vi "27-type_type.vi"(3 "this":i32, 4 "count in":i32, 5 "button":i32, 6 "Cluster":T1={"Auto1"=TRUE, "Auto2"=TRUE, "Rel1"=FALSE, "Rel2"=FALSE, "Filt1"=FALSE, "Filt2"=FALSE, "Rate"=enum."Slow", "Range1"=enum."10mV", "Range2"=enum."100mV", "Filt3"=FALSE, "Filt4"=FALSE, "Rel temp 1"=FALSE, "Analog1"=FALSE, "Analog2"=FALSE, "Analog temp 1"=FALSE, "Digital1"=FALSE, "Digital2"=FALSE, "Digital temp 1 "=FALSE, "Window1"=enum."None", "Window2"=enum."None", "Window temp 1"=enum."None", "RDGS1"="010", "RDGS2"="010", "RDGS temp 1"="010", "Type_type1"=TRUE, "Type_type2"=TRUE, "Type_type temp 1"=TRUE, "LSync"=FALSE, "Unit"=enum."C", "Sens"=TRUE, "Type tcoupl"=enum."J", "Junc"=TRUE, "prevState"=0, "Rel temp 2"=FALSE, "Analog temp 2"=FALSE, "Digital temp 2"=FALSE, "Type_type temp 2"=TRUE, "RDGS temp 2"="010", "Window temp 2"=enum."None", "address"="0"}) -> (0 "next state":i32, 1 "count out":i32, 2 "Cluster 2":T1)   [LabVIEW 2017]
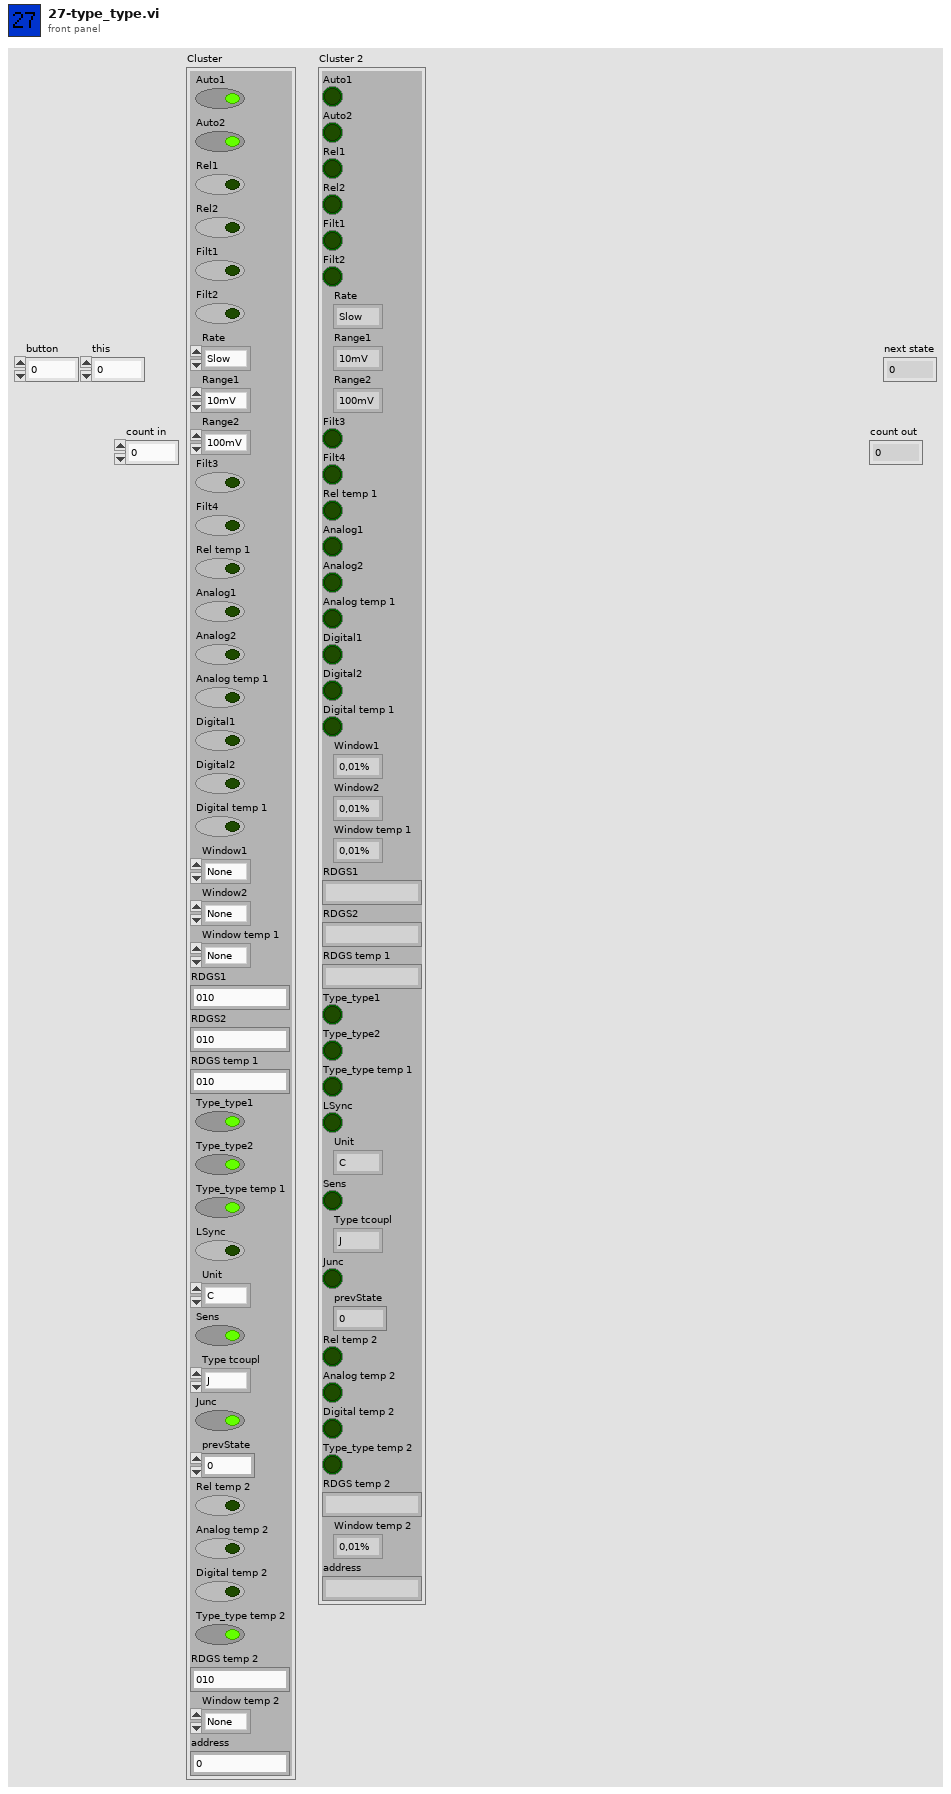
[diagram p1: front panel]
types:
  T1 = cluster{"Auto1":bool, "Auto2":bool, "Rel1":bool, "Rel2":bool, "Filt1":bool, "Filt2":bool, "Rate":enum16{"Slow", "Fast", "Med"}, "Range1":enum16{"10mV", "100mV", "1V", "10V", "100V"}, "Range2":enum16{"100mV", "1V", "10V"}, "Filt3":bool, "Filt4":bool, "Rel temp 1":bool, "Analog1":bool, "Analog2":bool, "Analog temp 1":bool, "Digital1":bool, "Digital2":bool, "Digital temp 1 ":bool, "Window1":enum16{"0,01%", "0,1%", "1%", "10%", "None"}, "Window2":enum16{"0,01%", "0,1%", "1%", "10%", "None"}, "Window temp 1":enum16{"0,01%", "0,1%", "1%", "10%", "None"}, "RDGS1":string, "RDGS2":string, "RDGS temp 1":string, "Type_type1":bool, "Type_type2":bool, "Type_type temp 1":bool, "LSync":bool, "Unit":enum16{"C", "K", "F"}, "Sens":bool, "Type tcoupl":enum16{"J", "K", "T", "E", "R", "S", "B", "N"}, "Junc":bool, "prevState":i32, "Rel temp 2":bool, "Analog temp 2":bool, "Digital temp 2":bool, "Type_type temp 2":bool, "RDGS temp 2":string, "Window temp 2":enum16{"0,01%", "0,1%", "1%", "10%", "None"}, "address":string}
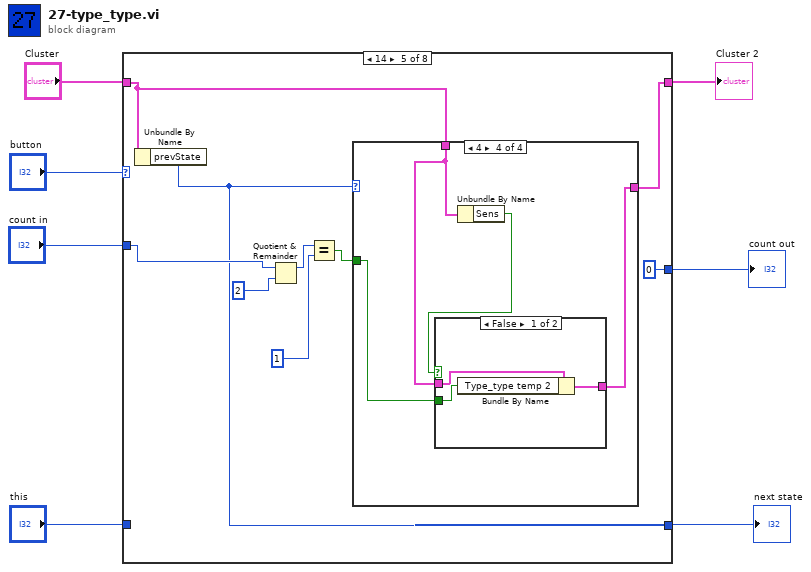
[diagram p0: block diagram]
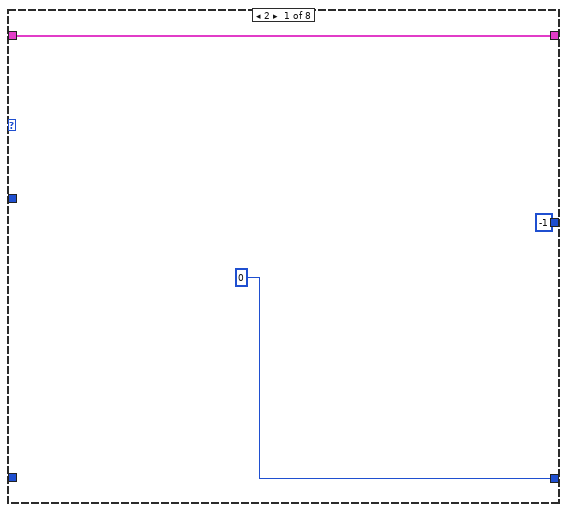
[diagram p2: hidden frame]
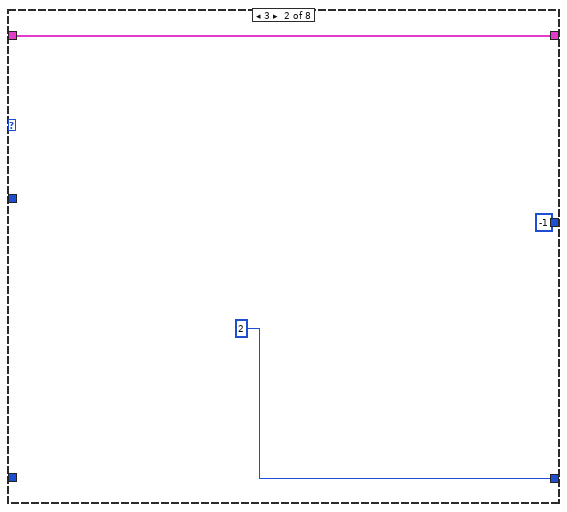
[diagram p3: hidden frame]
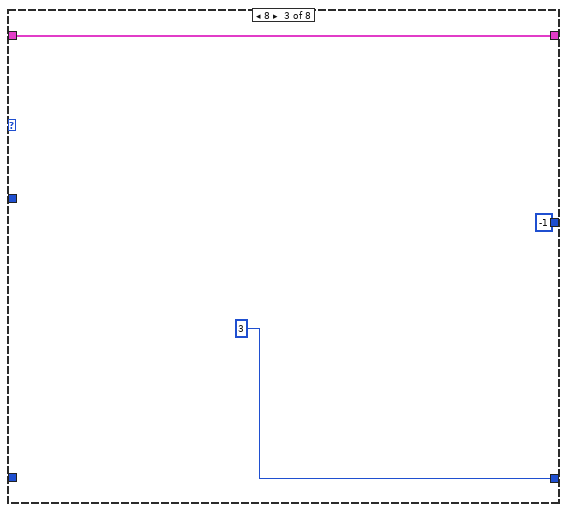
[diagram p4: hidden frame]
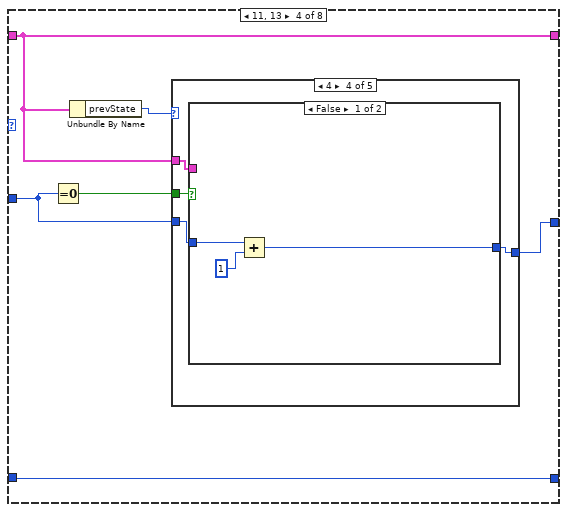
[diagram p5: hidden frame]
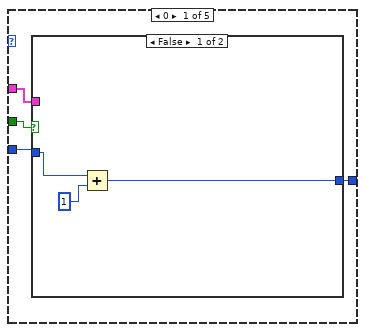
[diagram p6: hidden frame]
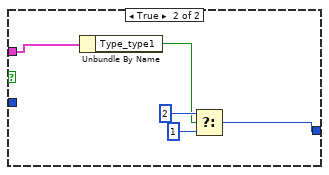
[diagram p7: hidden frame]
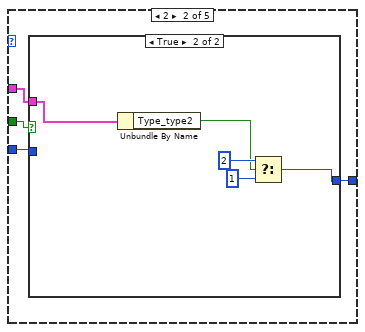
[diagram p8: hidden frame]
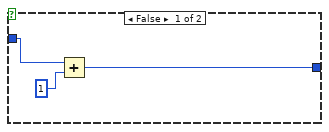
[diagram p9: hidden frame]
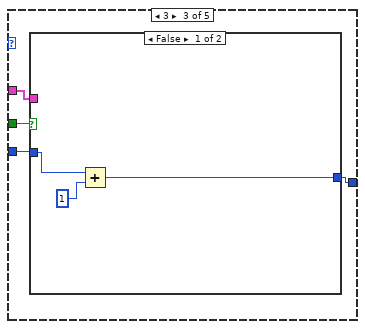
[diagram p10: hidden frame]
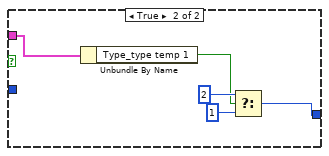
[diagram p11: hidden frame]
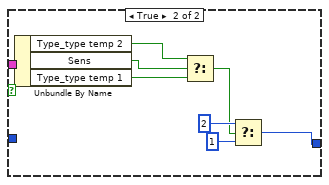
[diagram p12: hidden frame]
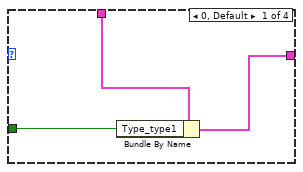
[diagram p14: hidden frame]
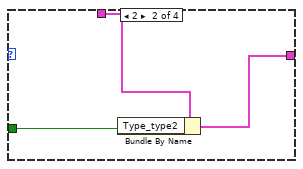
[diagram p15: hidden frame]
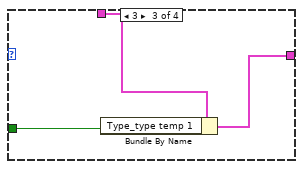
[diagram p16: hidden frame]
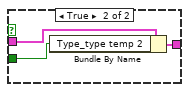
[diagram p17: hidden frame]
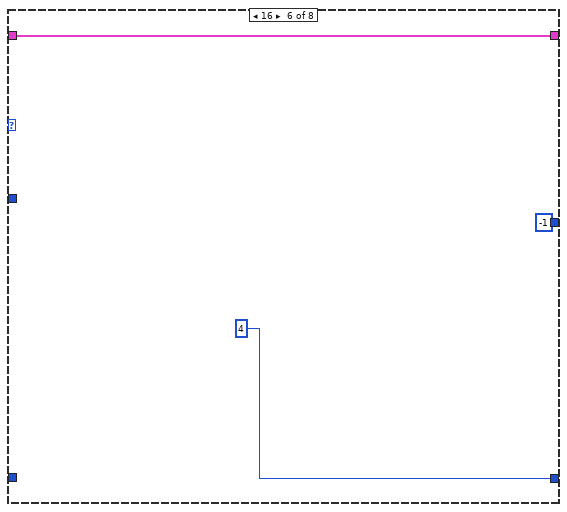
[diagram p18: hidden frame]
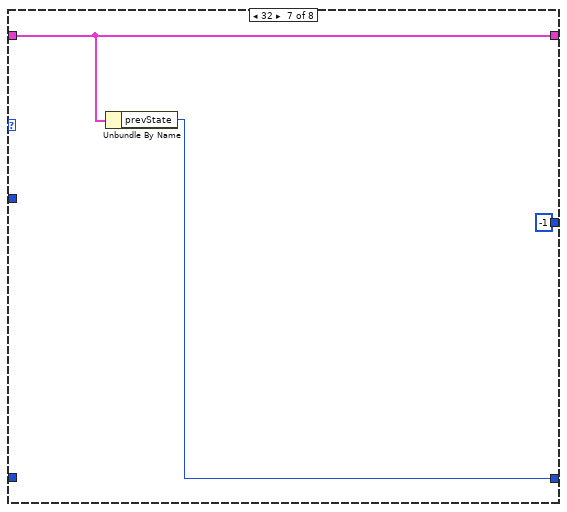
[diagram p19: hidden frame]
diagram:
  n1 = case shown="14" "button" {
    tunnel: [0 ("this") 2 3 w22 w75 4 w107 w110] -> w5
    tunnel: "this" -> [_ _ _ w22 _ _ _ w110]
    tunnel: "Cluster" -> [w10 w12 w15 w18 w78 w104 w108 w111]
    tunnel: [w10 w12 w15 w18 w77 w104 w108 w111] -> w4
    tunnel: "count in" -> [_ _ _ w19 w80 _ _ w109]
    tunnel: [-1 ("window in") -1 ("window in") -1 ("window in") w17 0 ("count in") -1 ("window in") -1 ("window in") w109] -> w2
    frame 2 {
    }
    frame 3 {
    }
    frame 8 {
    }
    frame 11, 13 {
      n2 = Equal To 0?(x=w19) -> (x = 0?=w20:bool)
      n3 = Unbundle By Name(w18) -> ("prevState"=w21:i32)
      n4 = case shown="4" w21 {
        tunnel: w20 -> [w25 w37 w49 w60 _]
        tunnel: w19 -> [w23 w35 w47 w59 w74]
        tunnel: w18 -> [w26 w38 w50 w61 _]
        tunnel: [w24 w36 w48 w62 w74] -> w17
        frame 0 {
          n5 = case shown="False" w25 {
            tunnel: [w28 w34] -> w24
            tunnel: w26 -> [_ w33]
            tunnel: w23 -> [w27 _]
            frame False {
              n6 = Add(x=w27, y=1) -> (x+y=w28:i32)
            }
            frame True {
              n7 = Unbundle By Name(w33) -> ("Type_type1"=w30:bool)
              n8 = Select(t=2, s=w30, f=1) -> (s? t:f=w34:i32)
            }
          }
        }
        frame 2 {
          n9 = case shown="True" w37 {
            tunnel: [w40 w46] -> w36
            tunnel: w38 -> [_ w45]
            tunnel: w35 -> [w39 _]
            frame False {
              n10 = Add(x=w39, y=1) -> (x+y=w40:i32)
            }
            frame True {
              n11 = Unbundle By Name(w45) -> ("Type_type2"=w42:bool)
              n12 = Select(t=2, s=w42, f=1) -> (s? t:f=w46:i32)
            }
          }
        }
        frame 3 {
          n13 = case shown="False" w49 {
            tunnel: [w52 w58] -> w48
            tunnel: w50 -> [_ w57]
            tunnel: w47 -> [w51 _]
            frame False {
              n14 = Add(x=w51, y=1) -> (x+y=w52:i32)
            }
            frame True {
              n15 = Unbundle By Name(w57) -> ("Type_type temp 1"=w54:bool)
              n16 = Select(t=2, s=w54, f=1) -> (s? t:f=w58:i32)
            }
          }
        }
        frame 4 {
          n17 = case shown="False" w60 {
            tunnel: [w64 w73] -> w62
            tunnel: w61 -> [_ w72]
            tunnel: w59 -> [w63 _]
            frame False {
              n18 = Add(x=w63, y=1) -> (x+y=w64:i32)
            }
            frame True {
              n19 = Unbundle By Name(w72) -> ("Type_type temp 2"=w68:bool, "Sens"=w69:bool, "Type_type temp 1"=w67:bool)
              n20 = Select(t=w68, s=w69, f=w67) -> (s? t:f=w66:bool)
              n21 = Select(t=2, s=w66, f=1) -> (s? t:f=w73:i32)
            }
          }
        }
        frame Default {
        }
      }
    }
    frame 14 {
      n22 = Unbundle By Name(w78) -> ("prevState"=w75:i32)
      n23 = Quotient & Remainder(x=w80, y=2) -> (x-y*floor(x/y)=w82:i32)  [unwired: 1 out]
      n24 = Equal?(x=w82, y=1 ("x")) -> (x = y?=w79:bool)
      n25 = case shown="4" w75 {
        tunnel: w79 -> [w86 w89 w92 w94]
        tunnel: w78 -> [w85 w87 w90 w95]
        tunnel: [w84 w88 w91 w93] -> w77
        frame 0, Default {
          n26 = Bundle By Name(cluster=w85, "Type_type1"=w86) -> (w84:T1)
        }
        frame 2 {
          n27 = Bundle By Name(cluster=w87, "Type_type2"=w89) -> (w88:T1)
        }
        frame 3 {
          n28 = Bundle By Name(cluster=w90, "Type_type temp 1"=w92) -> (w91:T1)
        }
        frame 4 {
          n29 = Unbundle By Name(w95) -> ("Sens"=w96:bool)
          n30 = case shown="False" w96 {
            tunnel: w95 -> [w98 w102]
            tunnel: w94 -> [w99 w101]
            tunnel: [w97 w100] -> w93
            frame False {
              n31 = Bundle By Name(cluster=w98, "Type_type temp 2"=w99) -> (w97:T1)
            }
            frame True {
              n32 = Bundle By Name(cluster=w102, "Type_type temp 2"=w101) -> (w100:T1)
            }
          }
        }
      }
    }
    frame 16 {
    }
    frame 32 {
      n33 = Unbundle By Name(w108) -> ("prevState"=w107:i32)
    }
    frame Default {
    }
  }
  "next state" <- w5
  "count out" <- w2
  "Cluster 2" <- w4
